vi "PipBoy_Fmt_PaddPagesWithEmptyPictures.vi"(8 "error in":errorcluster, 9 "Icons by page":i32=8, 10 "function icons":T1[](array[typedef]), 11 "function names":string[](array[string])) -> (0 "error out":errorcluster, 2 "function icons 2":T1[](array[typedef]), 3 "function names 2":string[](array[string]))   [LabVIEW 2014]
uses:
  <vilib>/picture/picture.llb/imagedata.ctl
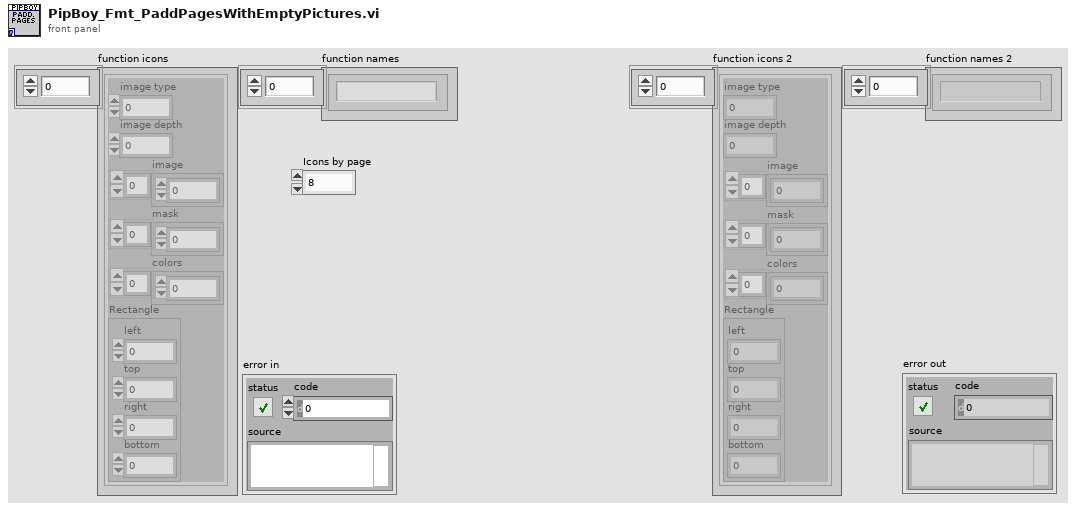
[diagram p1: front panel]
types:
  T1 = typedef "imagedata.ctl" = cluster{"image type":i32, "image depth":i32, "image":u8[], "mask":u8[], "colors":u32[], "Rectangle":cluster{"left":i16, "top":i16, "right":i16, "bottom":i16}}
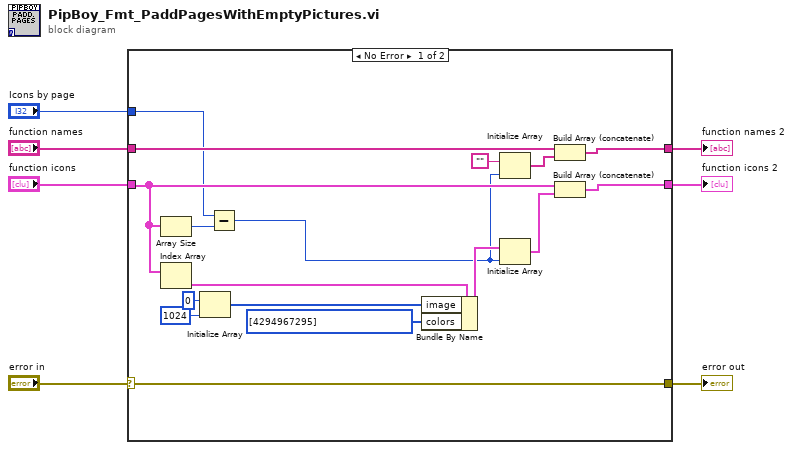
[diagram p0: block diagram]
diagram:
  n1 = case shown="No Error" "error in" {
    selector: "error in" -> [w24 w27]
    tunnel: [w24 w27] -> w6
    tunnel: [w19 w26] -> w5
    tunnel: "function icons" -> [w21 w26]
    tunnel: [w17 w25] -> w3
    tunnel: "function names" -> [w18 w25]
    tunnel: "Icons by page" -> [w10 _]
    frame No Error {
      n2 = Array Size(array=w21) -> (size(s)=w8:i32)
      n3 = Index Array(array=w21) -> (element=w23:T1)  [unwired: 1 in]
      n4 = Initialize Array(u8 0, 1024 ("dimension size")) -> (w13:u8[])
      n5 = Subtract(x=w10, y=w8) -> (x-y=w9:i32)
      n6 = Bundle By Name(cluster=w23, "image"=w13, "colors"=u32[] [4294967295]) -> (w22:T1)
      n7 = Initialize Array("", w9) -> (w16:string[])
      n8 = Initialize Array(w22, w9) -> (w20:T1[])
      n9 = Build Array (concatenate)(w18, w16) -> (w17:string[])
      n10 = Build Array (concatenate)(w21, w20) -> (w19:T1[])
    }
    frame Error {
    }
  }
  "function icons 2" <- w5
  "function names 2" <- w3
  "error out" <- w6
